vi "Simple TCP - Client - 1.vi"() -> ()   [LabVIEW 2015]
doc: "Demonstrates how to open a connection to an TCP server, read the data being sent, and display the data on a chart. This VI is designed to stop if the TCP connection is terminated."
uses:
  <vilib>/Platform/TimedLoop/XDataNode/timing_clust.ctl
  <vilib>/Platform/TimedLoop/XDataNode/nitl_modes.ctl
  <vilib>/Platform/TimedLoop/XDataNode/wakeup.ctl
  <vilib>/platform/TimedLoop/XDataNode/XDataNode.xnode
  <vilib>/Platform/TimedLoop/XDataNode/XDNodeRunTimeDep.lvlib
panel:
  out "i":i32
  out "Time":u32
  out "value":T1
  in  "Server Closed":string="The server VI closed the connection."
  in  "Stop":bool
  # "Overview: Demonstrates the use of the TCP functions to connect to a TCP server VI and receive data.\nInstructions:\n1. Ensure Simple TCP - Server.vi is already running.\n2. Run the VI.\n3. Click Stop to stop the VI. Note that if you stop the server VI, this VI will stop automatically."
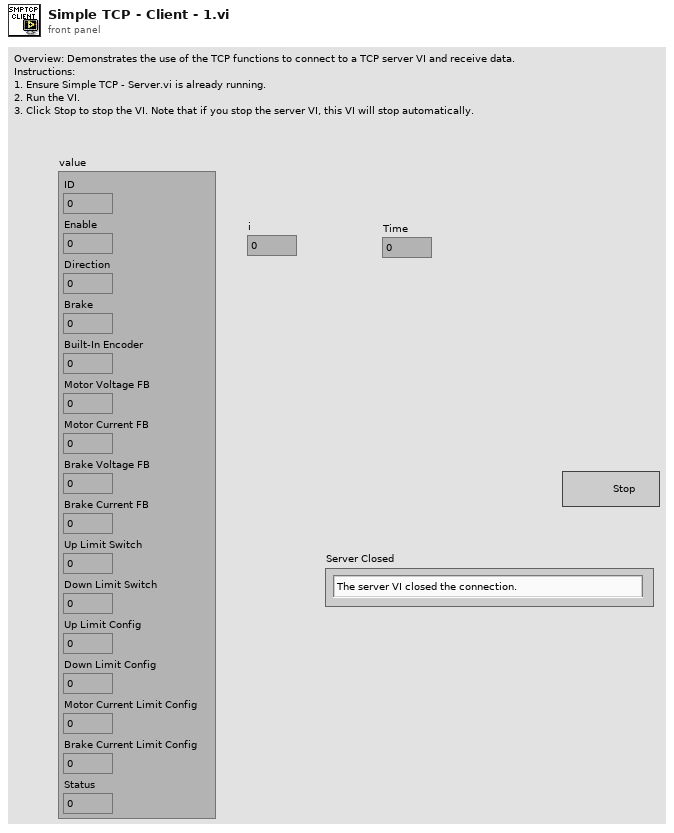
[diagram p1: front panel]
types:
  T1 = cluster{"ID":dbl, "Enable":dbl, "Direction":dbl, "Brake":dbl, "Built-In Encoder":dbl, "Motor Voltage FB":dbl, "Motor Current FB":dbl, "Brake Voltage FB":dbl, "Brake Current FB":dbl, "Up Limit Switch":dbl, "Down Limit Switch":dbl, "Up Limit Config":dbl, "Down Limit Config":dbl, "Motor Current Limit Config":dbl, "Brake Current Limit Config":dbl, "Status":dbl}
  T2 = typedef "XDNodeRunTimeDep.lvlib/timing_clust.ctl" = cluster{"Expected End [f-1]":u64, "Actual End [f-1]":u64, "Finished Late? [f-1]":bool, "Expected End [i-1]":u64, "Actual End [i-1]":u64, "Finished Late? [i-1]":bool, "Expected Start [i]":u64, "Actual Start [i]":u64, "Expected Start [f]":u64, "Actual Start [f]":u64, "Source Name":string, "Structure Name":string, "Period":i64, "Deadline":i64, "Offset":i64, "Start":i64, "Priority":i32, "Timeout":i32, "Mode":T3, "Wakeup Reason":T4, "Error":errorcluster, "Source Type":string, "Secondary Source Type":string, "Global End Time":u64, "Global Start Time":u64, "Frame Duration":u64, "Iteration Duration":u64, "Assigned CPU":i32, "I/O Scan Engine Mode":u32}
  T3 = typedef "XDNodeRunTimeDep.lvlib/nitl_modes.ctl" = enum32{"No Change", "Process missed periods, maintain original phase", "Discard missed periods, maintain original phase", "Process missed periods, ignore original phase", "Discard missed periods, ignore original phase"}
  T4 = typedef "XDNodeRunTimeDep.lvlib/wakeup.ctl" = enum32{"Normal", "Aborted", "Asynchronous wakeup", "Timing source error", "Timed loop error", "Timeout"}
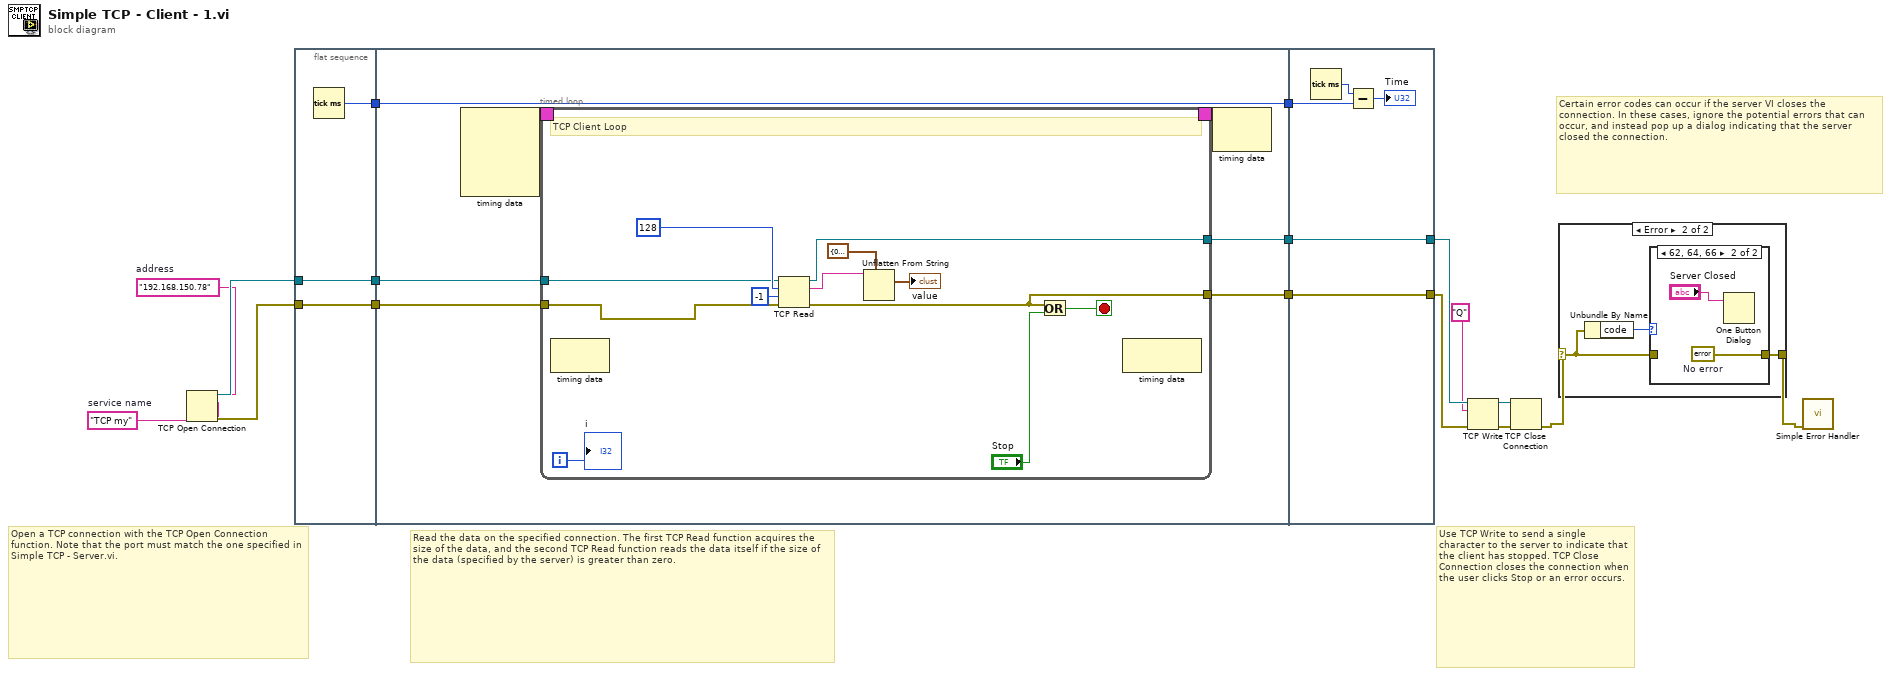
[diagram p0: block diagram]
diagram:
  w7 = "TCP my"  # service name
  w8 = "192.168.150.78"  # address
  # "Certain error codes can occur if the server VI closes the connection. In these cases, ignore the potential errors that can occur, and instead pop up a dialog indicating that the server closed the connection."
  # "Use TCP Write to send a single character to the server to indicate that the client has stopped. TCP Close Connection closes the connection when the user clicks Stop or an error occurs."
  # "Read the data on the specified connection. The first TCP Read function acquires the size of the data, and the second TCP Read function reads the data itself if the size of the data (specified by the server) is greater than zero."
  # "Open a TCP connection with the TCP Open Connection function. Note that the port must match the one specified in Simple TCP - Server.vi."
  n1 = TCP Open Connection(address=w8, remote port or service name=w7) -> (connection ID=w17:refnum<k5>, error out=w16:errorcluster)  [unwired: 3 in]
  n2 = flat-sequence {
    tunnel: w16 -> [w19]
    tunnel: w17 -> [w20]
    tunnel: [w20] -> w6
    tunnel: [w19] -> w5
    tunnel: [w18] -> w1
    tunnel: w6 -> [w21]
    tunnel: w5 -> [w22]
    tunnel: [w25] -> w4
    tunnel: [w24] -> w3
    tunnel: [w23] -> w2
    tunnel: w1 -> [w23]
    tunnel: [w47] -> w12
    tunnel: [w48] -> w14
    tunnel: w4 -> [w48]
    tunnel: w3 -> [w47]
    tunnel: w2 -> [w45]
    frame #0 {
      n3 = Tick Count (ms)() -> (millisecond timer value=w18:u32)
    }
    frame #1 {
      n4 = node-c288() -> (w27:T2)  [unwired: 4 in]
      n5 = timed-loop {
        tunnel: [w37] -> w25
        tunnel: [w36] -> w24
        timing: w27 -> [_]
        timing-out: [_] -> w26
        tunnel: w22 -> [w31]
        tunnel: w21 -> [w30]
        i -> [w28]
        stop <- w38 stop-if-true
        # "TCP Client Loop"
        n6 = node-c288() -> ()  [unwired: 1 in, 1 out]
        n7 = TCP Read(connection ID=w30, bytes to read=128, error in (no error)=w31, 9:-1 ("timeout ms (25000)")) -> (connection ID out=w37:refnum<k5>, data out=w33:string, error out=w36:errorcluster)  [unwired: 1 in]
        n8 = Unflatten From String(type=T1 {"ID"=0.0, "Enable"=0.0, "Direction"=0.0, "Brake"=0.0, "Built-In Encoder"=0.0, "Motor Voltage FB"=0.0, "Motor Current FB"=0.0, "Brake Voltage FB"=0.0, "Brake Current FB"=0.0, "Up Limit Switch"=0.0, "Down Limit Switch"=0.0, "Up Limit Config"=0.0, "Down Limit Config"=0.0, "Motor Current Limit Config"=0.0, "Brake Current Limit Config"=0.0, "Status"=0.0} ("MirrorCoverMotor"), binary string=w33) -> (value=→"value":T1)  [unwired: 3 in, 2 out]
        n9 = Or(x=w36, y="Stop") -> (x .or. y?=w38:bool)
        n10 = node-c288() -> ()  [unwired: 1 in, 1 out]
        "i" <- w28
      }
      n11 = node-c288(w26) -> ()  [unwired: 1 out]
    }
    frame #2 {
      n12 = Tick Count (ms)() -> (millisecond timer value=w46:u32)
      n13 = Subtract(x=w46, y=w45) -> (x-y=→"Time":u32)
    }
  }
  n14 = TCP Write(connection ID=w14, data in="Q", error in (no error)=w12) -> (connection ID out=w15:refnum<k5>, error out=w13:errorcluster)  [unwired: 2 out]
  n15 = TCP Close Connection(connection ID=w15, error in (no error)=w13) -> (error out=w10:errorcluster)  [unwired: 1 in, 1 out]
  n16 = case shown="Error" w10 {
    selector: w10 -> [w49 w51]
    tunnel: [w49 w50] -> w9
    frame No Error {
    }
    frame Error {
      n17 = Unbundle By Name(w51) -> ("code"=w52:i32)
      n18 = case shown="62, 64, 66" w52 {
        tunnel: w51 -> [w53 _]
        tunnel: [w53 w55] -> w50
        frame Default {
        }
        frame 62, 64, 66 {
          w55 = errorcluster {"status"=FALSE, "code"=0, "source"=""}  # No error
          n19 = One Button Dialog(message="Server Closed") -> ()  [unwired: 1 in, 1 out]
        }
      }
    }
  }
  n20 = call <vilib>:"Simple Error Handler.vi"("error in (no error)"=w9) -> ()  [unwired: 4 in, 5 out]
